vi "Create.vi"(8 "error in (no error)":errorcluster, 10 "MsgQ":refnum<class "MessageQ.lvclass">) -> (0 "error out":errorcluster, 3 "HardwareHTTPController out":refnum<class "HardwareHTTPController.lvclass">)   [LabVIEW 2020, in "Volatus.lvlib" / "HardwareHTTPController.lvclass"]
uses:
  HardwareHTTPController.lvclass
  HardwareHTTPController.lvclass/HardwareHTTPController.ctl
  MessageQ/MessageQ.lvclass
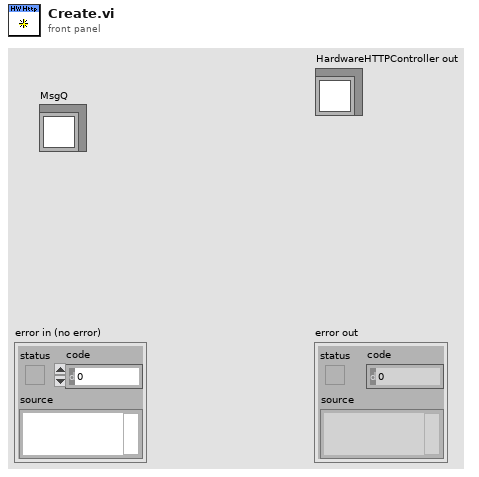
[diagram p1: front panel]
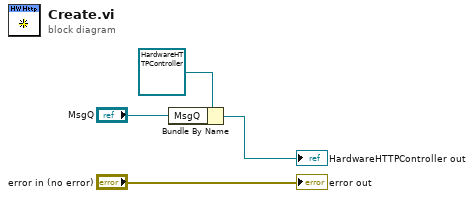
[diagram p0: block diagram]
diagram:
  n1 = Bundle By Name(cluster=refnum<class "HardwareHTTPController.lvclass"> refnum ("HardwareHTTPController in"), "MsgQ"="MsgQ") -> (→"HardwareHTTPController out":refnum<class "HardwareHTTPController.lvclass">)
  "error out" <- "error in (no error)"
